vi "Read Dashboard Variables.vi"() -> ()   [LabVIEW 2018]
uses:
  <vilib>/Rock Robotics/Network Tables/NT Read Number.vi
  Framework/Robot Global Data.vi
panel:
  out "Hatch Mover Scale":dbl=1.0 min=0.0 max=1.0 step=0.1
  out "Elevator Scale":dbl=1.0 min=0.0 max=1.0 step=0.1
  out "Autonomous Wait":u32=10
  out "Hatch Mover Duration":dbl=3.0
  out "Hatch Mover Setpoint":dbl=1.0
  out "SlowModeSettings":i32=2
  out "MaxSpeedSlow":dbl=0.4
  out "SlowRate":dbl=1.0
  out "MaxTurnSlow":dbl=0.55
  out "MaxTurnRateSlow":dbl=20.0
  out "Cargo Stop Current":dbl=10.0
  out "Cargo Hold Duration":dbl=1.0
  out "Cheezy Drive Mode":u32=2
  out "Cargo Setpoint":dbl=1.0 min=0.0 max=1.0 step=0.1
  out "Elevator Duration":dbl=2.0
  out "Elevator Setpoint":dbl=1.0 min=0.0 max=1.0 step=0.1
  out "Pivot Right Setpoint":dbl=0.3 min=0.0 max=1.0 step=0.1
  out "Pivot Left Setpoint":dbl=0.3 min=0.0 max=1.0 step=0.1
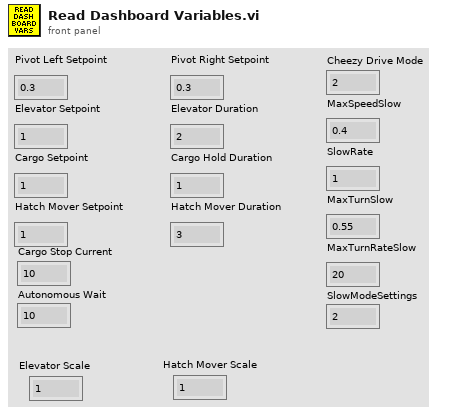
[diagram p1: front panel]
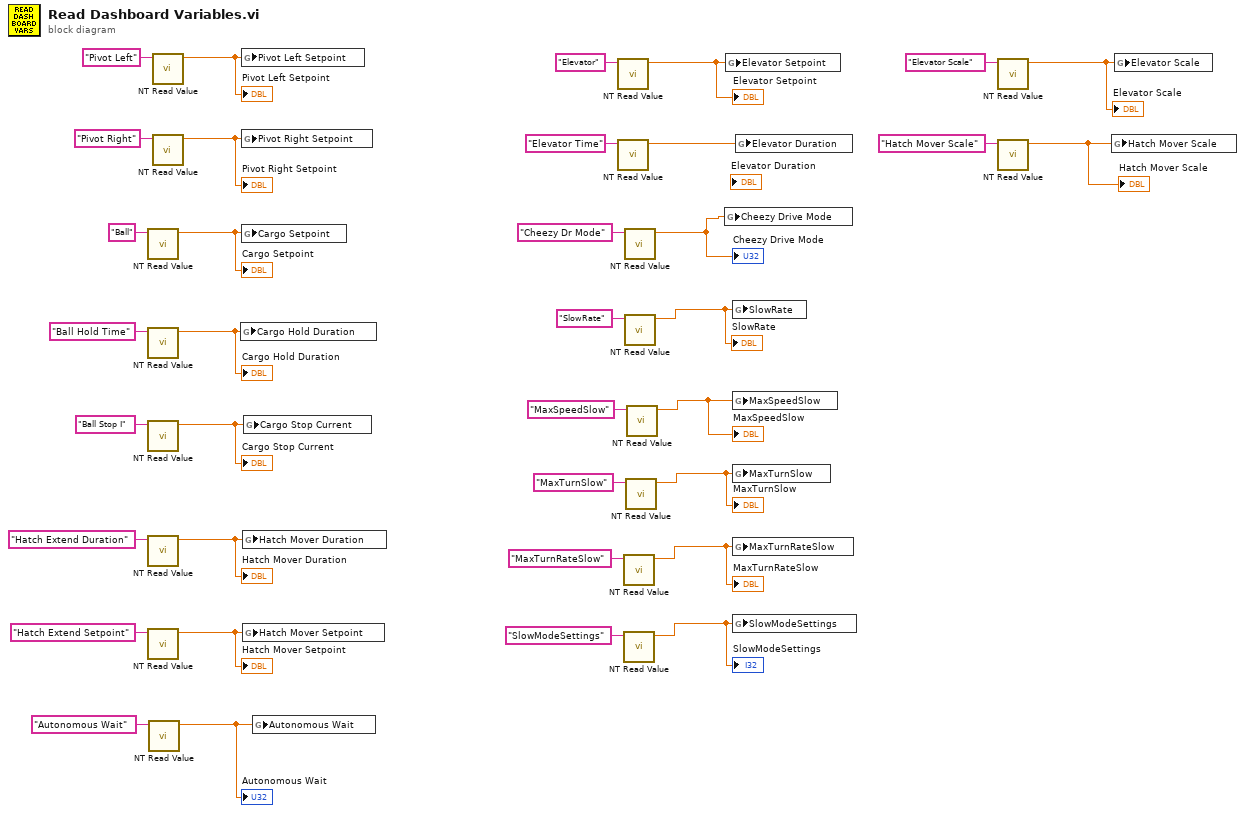
[diagram p0: block diagram]
diagram:
  n1 = call-poly <vilib>:"NT Read Value.vi"("Name"="Ball") -> ("Numeric"=w18:dbl)  [unwired: 9 in, 1 out]
  "Cargo Setpoint" <- w18
  n2 = call-poly <vilib>:"NT Read Value.vi"("Name"="Ball Hold Time") -> ("Numeric"=w17:dbl)  [unwired: 9 in, 1 out]
  "Cargo Hold Duration" <- w17
  n3 = call-poly <vilib>:"NT Read Value.vi"("Name"="Ball Stop I") -> ("Numeric"=w16:dbl)  [unwired: 9 in, 1 out]
  "Cargo Stop Current" <- w16
  n4 = call-poly <vilib>:"NT Read Value.vi"("Name"="Hatch Extend Duration") -> ("Numeric"=w15:dbl)  [unwired: 9 in, 1 out]
  "Hatch Mover Duration" <- w15
  n5 = call-poly <vilib>:"NT Read Value.vi"("Name"="Hatch Extend Setpoint") -> ("Numeric"=w14:dbl)  [unwired: 9 in, 1 out]
  "Hatch Mover Setpoint" <- w14
  n6 = call-poly <vilib>:"NT Read Value.vi"("Name"="Autonomous Wait") -> ("Numeric"=w5:dbl)  [unwired: 9 in, 1 out]
  "Autonomous Wait" <- w5
  n7 = call-poly <vilib>:"NT Read Value.vi"("Name"="Pivot Left") -> ("Numeric"=w20:dbl)  [unwired: 9 in, 1 out]
  "Pivot Left Setpoint" <- w20
  n8 = call-poly <vilib>:"NT Read Value.vi"("Name"="Pivot Right") -> ("Numeric"=w19:dbl)  [unwired: 9 in, 1 out]
  "Pivot Right Setpoint" <- w19
  n9 = global write "Robot Global Data.vi" "Cargo Hold Duration"(w17) -> ()
  n10 = global write "Robot Global Data.vi" "Pivot Left Setpoint"(w20) -> ()
  n11 = global write "Robot Global Data.vi" "Pivot Right Setpoint"(w19) -> ()
  n12 = global write "Robot Global Data.vi" "Cargo Setpoint"(w18) -> ()
  n13 = global write "Robot Global Data.vi" "Hatch Mover Duration"(w15) -> ()
  n14 = global write "Robot Global Data.vi" "Hatch Mover Setpoint"(w14) -> ()
  n15 = global write "Robot Global Data.vi" "Cargo Stop Current"(w16) -> ()
  n16 = global write "Robot Global Data.vi" "Autonomous Wait"(w5) -> ()
  n17 = call-poly <vilib>:"NT Read Value.vi"("Name"="Elevator") -> ("Numeric"=w7:dbl)  [unwired: 9 in, 1 out]
  "Elevator Setpoint" <- w7
  n18 = call-poly <vilib>:"NT Read Value.vi"("Name"="Elevator Time") -> ("Numeric"=w30:dbl)  [unwired: 9 in, 1 out]
  n19 = call-poly <vilib>:"NT Read Value.vi"("Name"="MaxTurnRateSlow") -> ("Numeric"=w9:dbl)  [unwired: 9 in, 1 out]
  "MaxTurnRateSlow" <- w9
  n20 = call-poly <vilib>:"NT Read Value.vi"("Name"="SlowModeSettings") -> ("Numeric"=w8:dbl)  [unwired: 9 in, 1 out]
  "SlowModeSettings" <- w8
  n21 = call-poly <vilib>:"NT Read Value.vi"("Name"="Cheezy Dr Mode") -> ("Numeric"=w13:dbl)  [unwired: 9 in, 1 out]
  "Cheezy Drive Mode" <- w13
  n22 = call-poly <vilib>:"NT Read Value.vi"("Name"="SlowRate") -> ("Numeric"=w12:dbl)  [unwired: 9 in, 1 out]
  "SlowRate" <- w12
  n23 = call-poly <vilib>:"NT Read Value.vi"("Name"="MaxTurnSlow") -> ("Numeric"=w10:dbl)  [unwired: 9 in, 1 out]
  "MaxTurnSlow" <- w10
  n24 = call-poly <vilib>:"NT Read Value.vi"("Name"="MaxSpeedSlow") -> ("Numeric"=w11:dbl)  [unwired: 9 in, 1 out]
  "MaxSpeedSlow" <- w11
  n25 = global write "Robot Global Data.vi" "Cheezy Drive Mode"(w13) -> ()
  n26 = global write "Robot Global Data.vi" "Elevator Setpoint"(w7) -> ()
  n27 = global write "Robot Global Data.vi" "SlowRate"(w12) -> ()
  n28 = global write "Robot Global Data.vi" "MaxSpeedSlow"(w11) -> ()
  n29 = global write "Robot Global Data.vi" "MaxTurnSlow"(w10) -> ()
  n30 = global write "Robot Global Data.vi" "MaxTurnRateSlow"(w9) -> ()
  n31 = global write "Robot Global Data.vi" "SlowModeSettings"(w8) -> ()
  n32 = global write "Robot Global Data.vi" "Elevator Duration"(w30) -> ()
  n33 = call-poly <vilib>:"NT Read Value.vi"("Name"="Elevator Scale") -> ("Numeric"=w2:dbl)  [unwired: 9 in, 1 out]
  "Elevator Scale" <- w2
  n34 = call-poly <vilib>:"NT Read Value.vi"("Name"="Hatch Mover Scale") -> ("Numeric"=w1:dbl)  [unwired: 9 in, 1 out]
  "Hatch Mover Scale" <- w1
  n35 = global write "Robot Global Data.vi" "Hatch Mover Scale"(w1) -> ()
  n36 = global write "Robot Global Data.vi" "Elevator Scale"(w2) -> ()
